vi "Car Wash Main.vi"() -> ()   [LabVIEW 2018]
doc: "The Car Wash Main VI is the main application that will provide the user with the interactive interface to initiate a car wash. This VI will utilize JKI state machine to incorperate each state of the car wash."
uses:
  Controls/Wash Option.ctl
  Controls/Wash Option Indicators.ctl
  Controls/Car Position.ctl
panel:
  in  "Car Position Slider":T1 scale=0.0..4.0
  out "Elapse Time":dbl format="%#_3g"
  in  "Stop Program":bool
  out "Wash Entry":bool
  out "Car Wash Indicators":T2
  in  "Start":bool
  in  "Wash Option":T3
  # "Entry Console"
  # "Car Wash Display"
  # "Pre-Soak\nH-P Wash\nL-P Waxx\nSpot Free Rinse"
  # "Underbody Wash\nBug Remover"
  # "Tire Shine\nAir Dry"
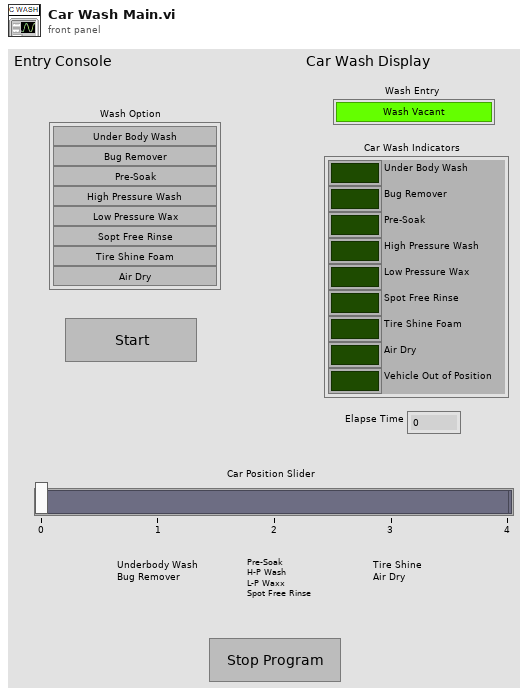
[diagram p1: front panel]
types:
  T1 = typedef "Car Position.ctl" = i32
  T2 = typedef "Wash Option Indicators.ctl" = cluster{"Under Body Wash":bool, "Bug Remover":bool, "Pre-Soak":bool, "High Pressure Wash":bool, "Low Pressure Wax":bool, "Spot Free Rinse":bool, "Tire Shine Foam":bool, "Air Dry":bool, "Vehicle Out of Position":bool}
  T3 = typedef "Wash Option.ctl" = cluster{"Under Body Wash":bool, "Bug Remover":bool, "Pre-Soak":bool, "High Pressure Wash":bool, "Low Pressure Wax":bool, "Spot Free Rinse":bool, "Tire Shine Foam":bool, "Air Dry":bool}
  T4 = enum32{"Invalid", "Standard", "Closed", "Hidden", "Minimized", "Maximized"}
  T5 = enum32{"invalid app kind", "Development System", "Run Time System", "Student Edition", "Embedded LabVIEW", "Evaluation", "Custom"}
  T6 = cluster{"Core":cluster{"Current VI Reference":refnum<vi>, "Close Panel on Exit?":bool}, "Current Car Wash Remaining":bool[], "Car Current Position":T1, "Current Elapse Time":dbl, "Start Time":timestamp, "Start Wash":bool, "Current Wash Index":i32}
  T7 = cluster{"Current VI Reference":refnum<vi>, "Close Panel on Exit?":bool}
  T8 = enum8{"Enabled", "Disabled", "Disabled and Grayed Out"}
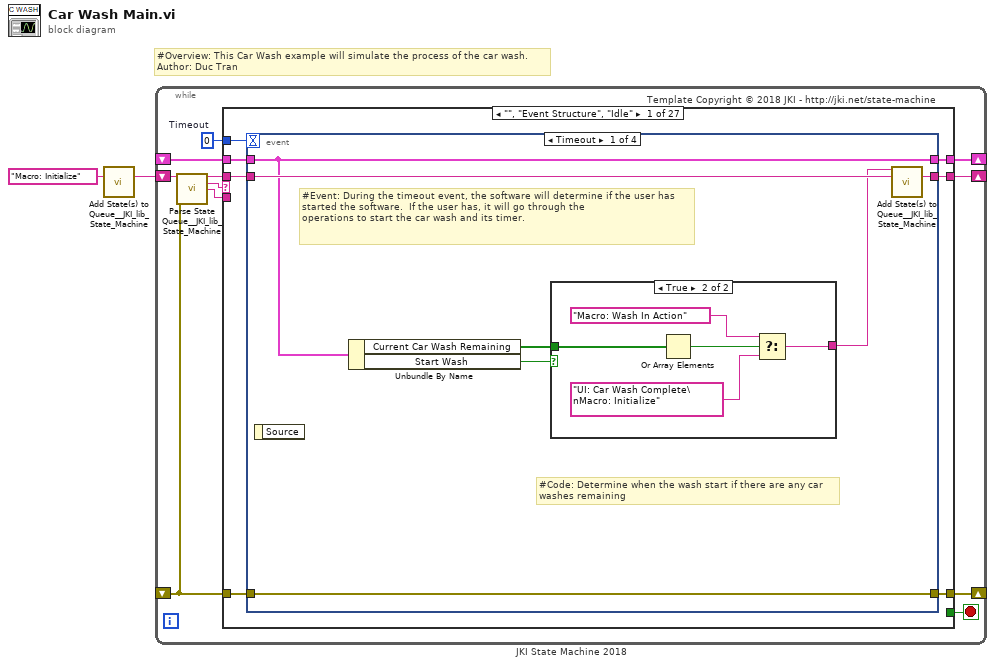
[diagram p0: block diagram]
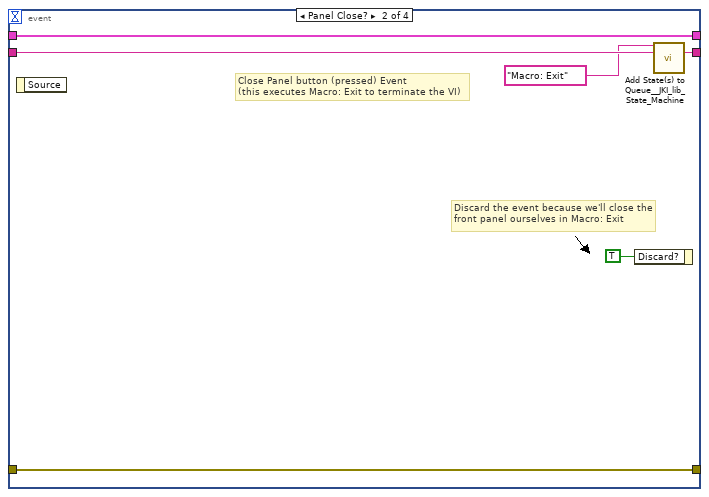
[diagram p3: hidden frame]
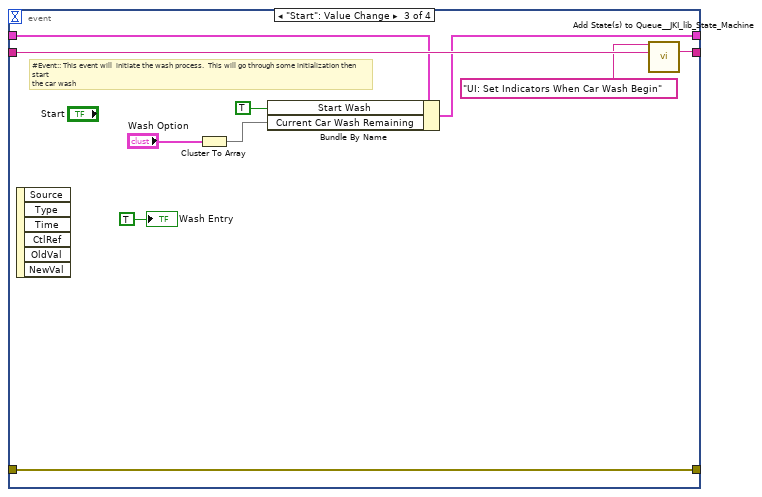
[diagram p4: hidden frame]
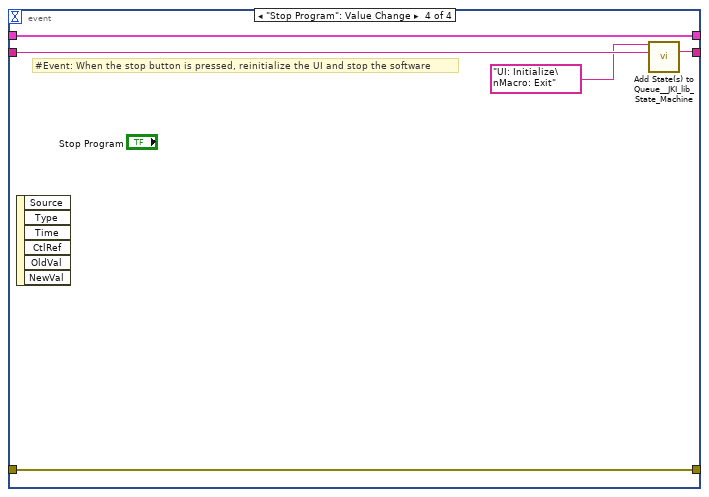
[diagram p5: hidden frame]
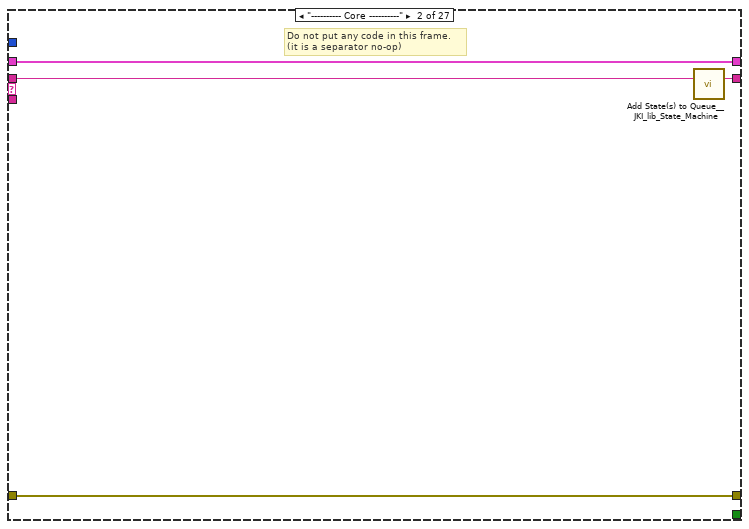
[diagram p6: hidden frame]
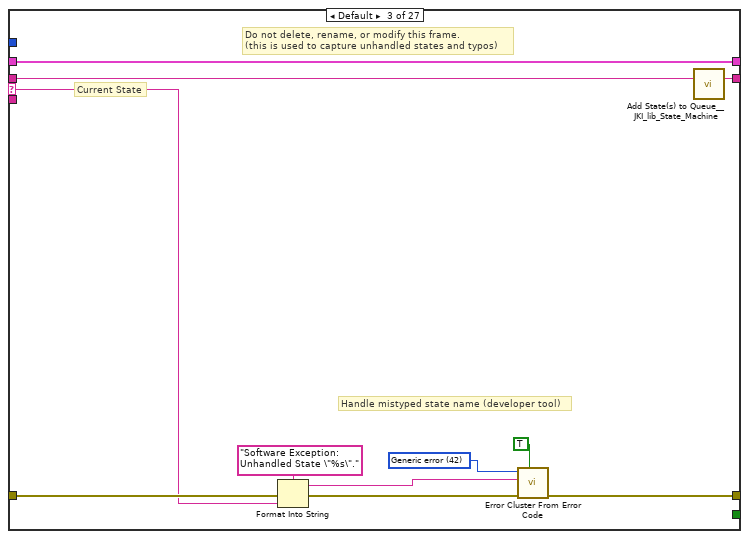
[diagram p7: hidden frame]
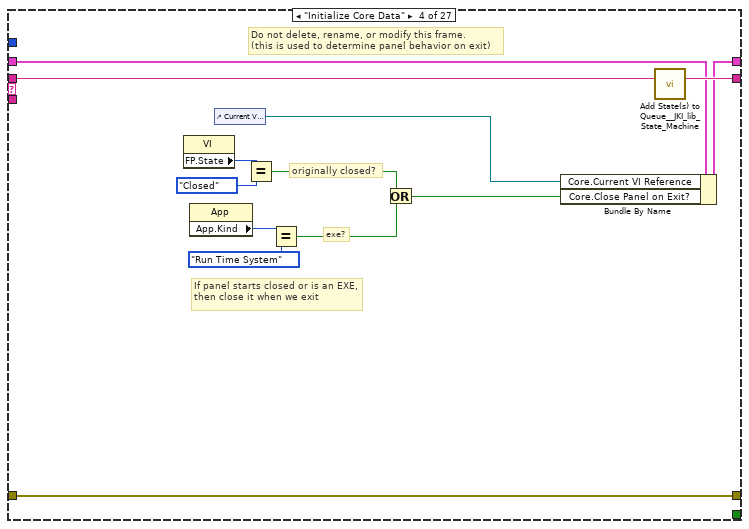
[diagram p8: hidden frame]
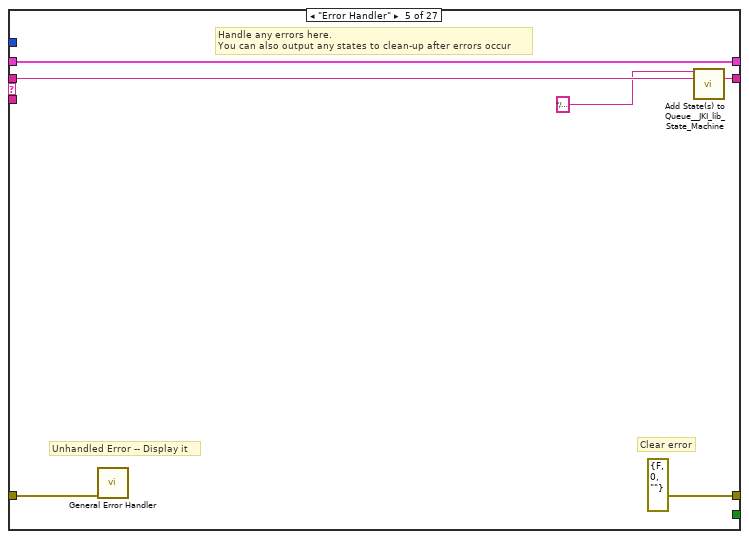
[diagram p9: hidden frame]
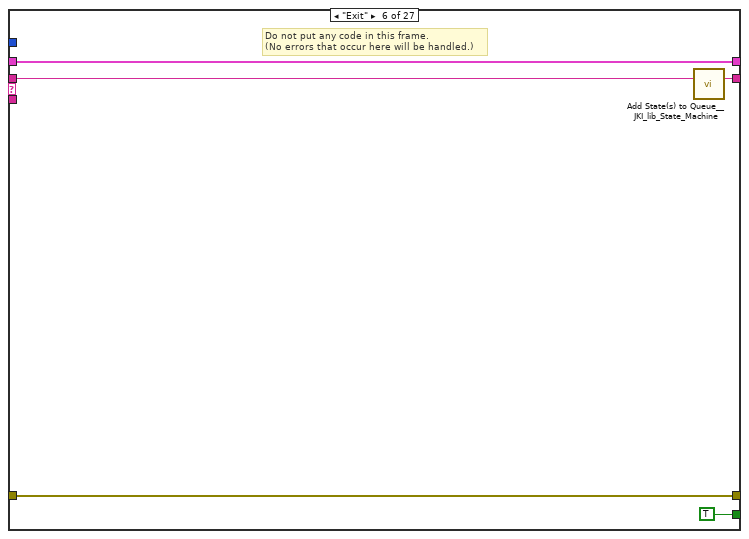
[diagram p10: hidden frame]
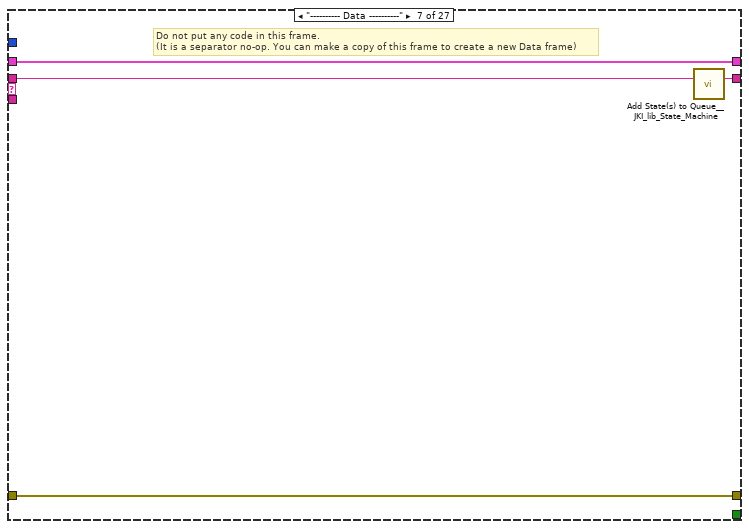
[diagram p11: hidden frame]
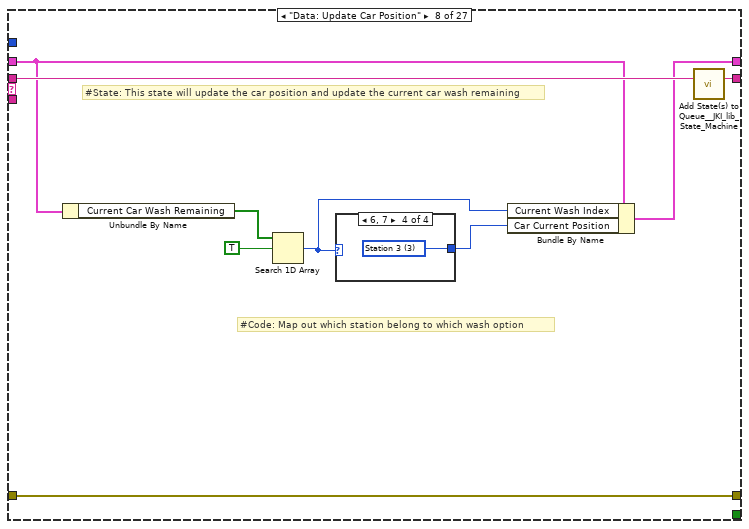
[diagram p12: hidden frame]
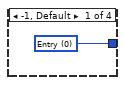
[diagram p13: hidden frame]
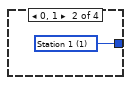
[diagram p14: hidden frame]
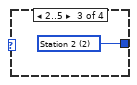
[diagram p15: hidden frame]
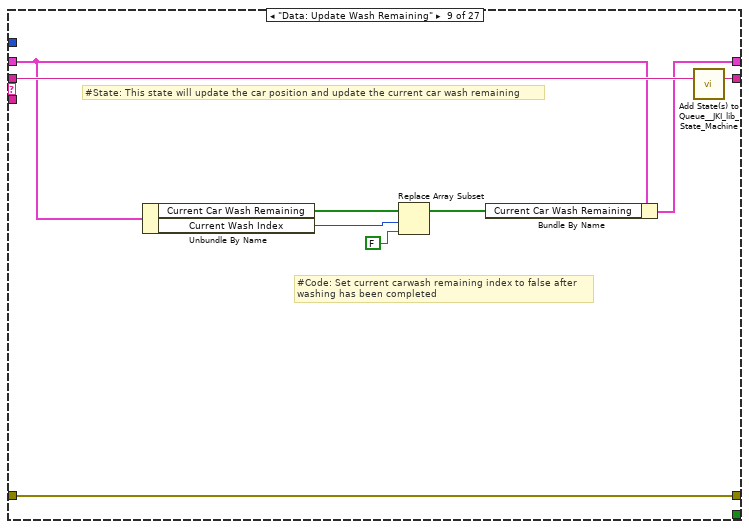
[diagram p16: hidden frame]
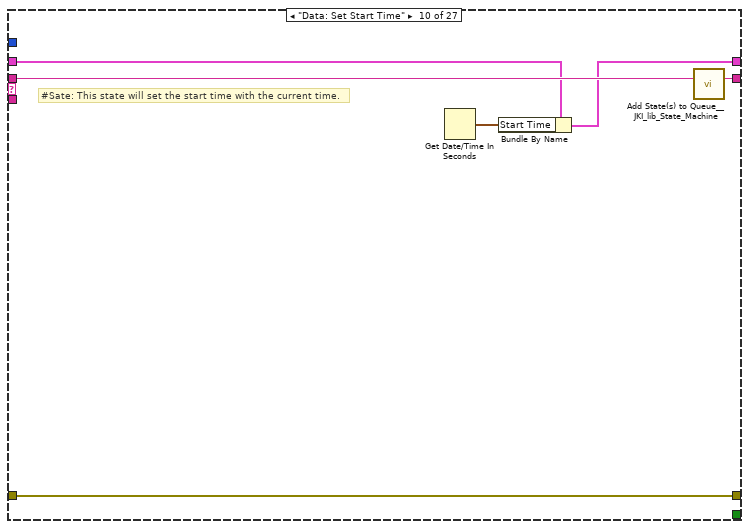
[diagram p17: hidden frame]
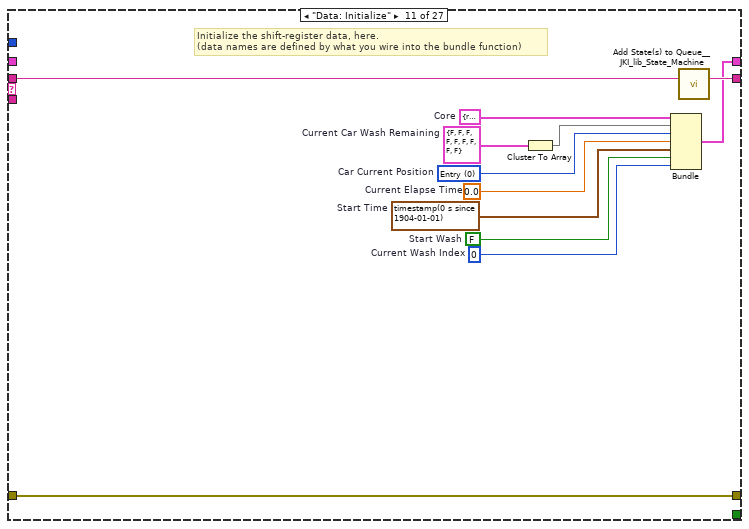
[diagram p18: hidden frame]
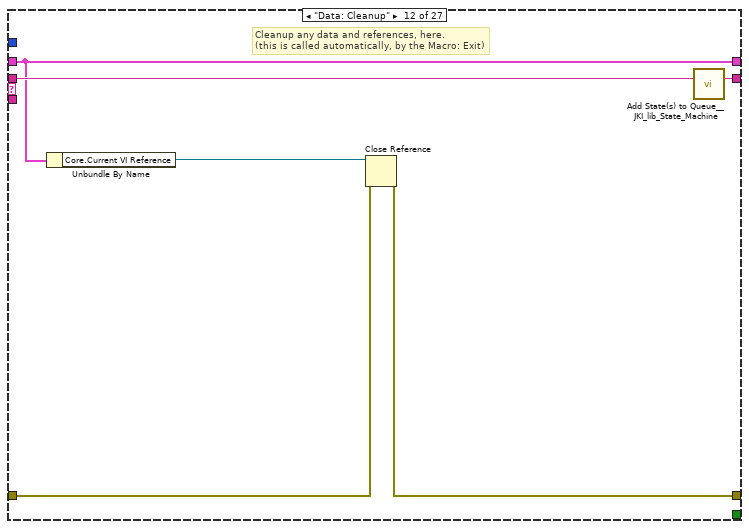
[diagram p19: hidden frame]
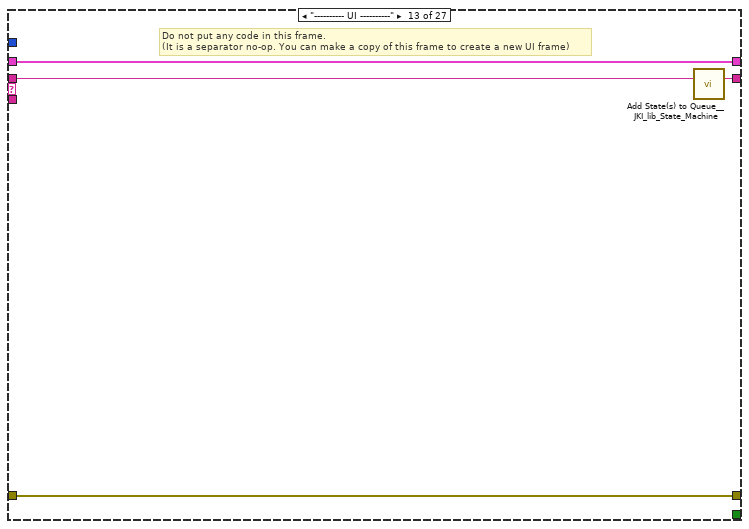
[diagram p20: hidden frame]
diagram:
  # "#Overview: This Car Wash example will simulate the process of the car wash.\nAuthor: Duc Tran"
  n1 = call <vilib>:"Add State(s) to Queue__JKI_lib_State_Machine.vi"("State(s) in (\"\")"="Macro: Initialize") -> ("States Out"=w1:string)  [unwired: 14 in]
  n2 = while "JKI State Machine 2018" {
    shift-right: [w6] -> _
    shift-left: _ -> [w5]
    shift-right: [w9] -> _
    shift-left: _ -> [w3]
    shift-right: [w8] -> _
    shift-left: w1 -> [w10]
    stop <- w7 stop-if-true
    w4 = 0  # Timeout
    # "Template Copyright © 2018 JKI - http://jki.net/state-machine"
    n3 = call <vilib>:"Parse State Queue__JKI_lib_State_Machine.vi"("State Queue"=w10, "Error In (no error)"=w3) -> ("Remaining States"=w12:string, "Current State"=w13:string, "Arguments"=w11:string)  [unwired: 11 in]
    n4 = case shown="\"\", \"Event Structure\", \"Idle\"" w13 {
      selector: w13 -> [_ _ w58 _ _ _ _ _ _ _ _ _ _ _ _ _ _ _ _ _ _ _ _ _ _ _ _]
      tunnel: w12 -> [w20 w57 w62 w81 w87 w92 w96 w105 w118 w124 w136 w142 w146 w149 w172 w179 w185 w200 w206 w217 w286 w291 w296 w306 w310 w320 w340]
      tunnel: w11 -> [_ _ _ _ _ _ _ _ _ _ _ _ _ _ _ _ _ _ w201 w211 _ _ _ _ _ _ _]
      tunnel: w5 -> [w18 w54 w60 w74 w84 w90 w93 w100 w115 w121 _ w138 w143 w150 w171 w177 w186 w198 w204 w213 w283 w288 w293 w303 w307 w317 w333]
      tunnel: [w17 w55 w64 w78 errorcluster {"status"=FALSE, "code"=0, "source"=""} ("error out") w89 w94 w103 w116 w122 w133 w139 w144 w151 w173 w180 w181 w189 w202 w214 w284 w289 w294 w304 w308 w318 w338] -> w9
      tunnel: w3 -> [w16 w55 w63 w78 w83 w89 w94 w103 w116 w122 w133 w137 w144 w151 w173 w180 w182 w194 w203 w215 w284 w289 w294 w304 w308 w318 w338]
      tunnel: [w19 w56 w61 w80 w86 w91 w95 w104 w117 w123 w135 w141 w145 w149 w172 w179 w185 w199 w205 w216 w285 w290 w295 w305 w309 w319 w339] -> w8
      tunnel: [_ _ _ _ _ TRUE _ _ _ _ _ _ _ _ _ _ _ _ _ _ _ _ _ _ _ _ _] -> w7
      tunnel: [w15 w54 w60 w79 w84 w90 w93 w99 w114 w120 w134 w138 w143 w150 w171 w175 w186 w198 w204 w213 w283 w288 w293 w303 w307 w317 w331] -> w6
      tunnel: w4 -> [w14 _ _ _ _ _ _ _ _ _ _ _ _ _ _ _ _ _ _ _ _ _ _ _ _ _ _]
      frame "", "Event Structure", "Idle" {
        n5 = event shown="[0] Timeout" {
          selector: _ -> [_ _ _ _]
          dyn-events: _ -> [_ _ _ _]
          timeout: w14 -> [_ _ _ _]
          tunnel: w20 -> [w27 w38 w48 w52]
          tunnel: [w26 w37 w47 w51] -> w19
          tunnel: w18 -> [w24 w35 w44 w53]
          tunnel: [w25 w36 w45 w49] -> w17
          tunnel: w16 -> [w25 w36 w45 w49]
          tunnel: [w24 w35 w42 w53] -> w15
          event Timeout {
            # "#Code: Determine when the wash start if there are any car\nwashes remaining"
            # "#Event: During the timeout event, the software will determine if the user has started the software.  If the user has, it will go through the\noperations to start the car wash and its timer."
            n6 = event-data() -> ()  [unwired: 1 in, 1 out]
            n7 = Unbundle By Name(w24) -> ("Current Car Wash Remaining"=w22:bool[], "Start Wash"=w23:bool)
            n8 = case shown="True" w23 {
              tunnel: w22 -> [_ w28]
              tunnel: [_ w30] -> w21
              frame False {
              }
              frame True {
                n9 = Or Array Elements(Boolean array=w28) -> (logical OR=w32:bool)
                n10 = Select(t="Macro: Wash In Action", s=w32, f="UI: Car Wash Complete\nMacro: Initialize") -> (s? t:f=w30:string)
              }
            }
            n11 = call <vilib>:"Add State(s) to Queue__JKI_lib_State_Machine.vi"("State(s) in Front (\"\")"=w21, "State(s) in (\"\")"=w27) -> ("States Out"=w26:string)  [unwired: 13 in]
          }
          event Panel Close? {
            # "Discard the event because we'll close the front panel ourselves in Macro: Exit"
            # "Close Panel button (pressed) Event\n(this executes Macro: Exit to terminate the VI)"
            n12 = event-data() -> ()  [unwired: 1 in, 1 out]
            n13 = event-data("Discard?"=TRUE) -> ()  [unwired: 1 in, 1 out]
            n14 = call <vilib>:"Add State(s) to Queue__JKI_lib_State_Machine.vi"("State(s) in Front (\"\")"="Macro: Exit", "State(s) in (\"\")"=w38) -> ("States Out"=w37:string)  [unwired: 13 in]
          }
          event "Start": Value Change {
            # "#Event:: This event will  initiate the wash process.  This will go through some initialization then start\nthe car wash"
            n15 = event-data() -> ()  [unwired: 1 in, 6 out]
            n16 = Cluster To Array(cluster="Wash Option") -> (array=w40:bool[])
            n17 = Bundle By Name(cluster=w44, "Start Wash"=TRUE, "Current Car Wash Remaining"=w40) -> (w42:T6)
            n18 = call <vilib>:"Add State(s) to Queue__JKI_lib_State_Machine.vi"("State(s) in Front (\"\")"="UI: Set Indicators When Car Wash Begin", "State(s) in (\"\")"=w48) -> ("States Out"=w47:string)  [unwired: 13 in]
            "Wash Entry" <- TRUE ("Wash Entry")
          }
          event "Stop Program": Value Change {
            # "#Event: When the stop button is pressed, reinitialize the UI and stop the software"
            n19 = event-data() -> ()  [unwired: 1 in, 6 out]
            n20 = call <vilib>:"Add State(s) to Queue__JKI_lib_State_Machine.vi"("State(s) in Front (\"\")"="UI: Initialize\nMacro: Exit", "State(s) in (\"\")"=w52) -> ("States Out"=w51:string)  [unwired: 13 in]
          }
        }
      }
      frame "---------- Core ----------" {
        # "Do not put any code in this frame.\n(it is a separator no-op)"
        n21 = call <vilib>:"Add State(s) to Queue__JKI_lib_State_Machine.vi"("State(s) in (\"\")"=w57) -> ("States Out"=w56:string)  [unwired: 14 in]
      }
      frame Default {
        w67 = 42 items=["No error", "Argument error", "Memory is full", "Out of zone", "End of file", "File already open", "Generic file I/O error", "File not found", "File permission error", "Disk is full", "Duplicate path", "Too many files open", "System feature not enabled", "Resource file not found", "Cannot add resource", "Resource not found", "Image not found", "Image memory error", "Pen does not exist", "Config type invalid", "Config token not found", "Config parse error", "Config memory error", "Bad external code format", "Bad external code offset", "External code not present", "Null window", "Destroy window error", "Null menu", "Print aborted", "Bad print record", "Print driver error", "Windows error during printing", "Memory error during printing", "Print dialog error", "Generic print error", "Invalid device refnum", "Device not found", "Device parameter error", "Device unit error", "Cannot open device", "Device call aborted", "Generic error", "Cancelled by user", "Object ID too low", "Object ID too high", "Object not in heap", "Unknown heap", "Unknown object (invalid DefProc)", "Unknown object (DefProc not in table)", "Message out of range", "Invalid (null) method", "Unknown message", "Manager call not supported", "Bad address", "Network operation in progress", "Network operation timed out", "Connection is busy", "Network attribute not supported", "Network error", "Address in use", "System out of memory", "Connection aborted", "Connection refused", "Not connected", "Already connected", "Connection closed", "Initialization error (interapplication manager)", "Bad occurrence", "Wait on unbound occurrence handler", "Occurrence queue overflow", "Datalog type conflict", "Unused", "Unrecognized type (interapplication manager)", "Memory corrupt", "Failed to make temporary DLL", "Old CIN version", "Drag socket not found", "Failed to load drop-object", "Failed to register OLE object", "Failed to release OLE object", "Format specifier type mismatch", "Unknown format specifier", "Too few format specifiers", "Too many format specifiers", "Scan failed", "Newer CIN version", "Error converting to variant", "Runtime menu error", "Password tampered", "Variant attribute not found", "Incompatible variant data type", "Event data is not available", "Event Store is not present", "Occurrence is not found", "Event Queue is not created", "Event info is not available", "Refnum passed is NULL", "Error retrieving Class GUID", "Error retrieving CoClass GUID", "Error retrieving TypeLib GUID.", "Bad built application magic bytes.", "Specific driver is different from the specific driver associated with the Logical Name.", "There is no session opened to the class driver.", "Max Error", "MAX - Error with config objects", "MAX - Error loading configuration", "MAX - Group not supported"]
        # "Current State"
        # "Do not delete, rename, or modify this frame.\n(this is used to capture unhandled states and typos)"
        # "Handle mistyped state name (developer tool)"
        n22 = Format Into String(format string="Software Exception: Unhandled State \"%s\"." ("message"), error in=w63, w58) -> (resulting string=w66:string, error out=w65:errorcluster)  [unwired: 1 in]
        n23 = call <vilib>:"Error Cluster From Error Code.vi"("show call chain? (False)"=TRUE, "error in (no error)"=w65, "error message (\"\")"=w66, "error code (0)"=w67) -> ("error out"=w64:errorcluster)  [unwired: 5 in]
        n24 = call <vilib>:"Add State(s) to Queue__JKI_lib_State_Machine.vi"("State(s) in (\"\")"=w62) -> ("States Out"=w61:string)  [unwired: 14 in]
      }
      frame "Initialize Core Data" {
        # "Do not delete, rename, or modify this frame.\n(this is used to determine panel behavior on exit)"
        # "originally closed?"
        # "exe?"
        # "If panel starts closed or is an EXE, then close it when we exit"
        n25 = property class="VI"() -> ("FP.State"=w71:T4)  [unwired: 2 in, 2 out]
        n26 = property class="App"() -> ("App.Kind"=w77:T5)  [unwired: 2 in, 2 out]
        n27 = control-ref of="Current VI Reference"() -> (w72:refnum<vi>)
        n28 = Equal?(x=w71, y=T4."Closed" ("Front Panel Window:State")) -> (x = y?=w69:bool)
        n29 = Equal?(x=w77, y=T5."Run Time System" ("Application:Kind")) -> (x = y?=w75:bool)
        n30 = Or(x=w69, y=w75) -> (x .or. y?=w73:bool)
        n31 = Bundle By Name(cluster=w74, "Core.Current VI Reference"=w72, "Core.Close Panel on Exit?"=w73) -> (w79:T6)
        n32 = call <vilib>:"Add State(s) to Queue__JKI_lib_State_Machine.vi"("State(s) in (\"\")"=w81) -> ("States Out"=w80:string)  [unwired: 14 in]
      }
      frame "Error Handler" {
        # "Unhandled Error -- Display it"
        # "Handle any errors here.\nYou can also output any states to clean-up after errors occur"
        # "Clear error"
        n33 = call <vilib>:"General Error Handler.vi"("error in (no error)"=w83) -> ()  [unwired: 10 in, 5 out]
        n34 = call <vilib>:"Add State(s) to Queue__JKI_lib_State_Machine.vi"("State(s) in Front (\"\")"="/* Post Error States", "State(s) in (\"\")"=w87) -> ("States Out"=w86:string)  [unwired: 13 in]
      }
      frame "Exit" {
        # "Do not put any code in this frame.\n(No errors that occur here will be handled.)"
        n35 = call <vilib>:"Add State(s) to Queue__JKI_lib_State_Machine.vi"("State(s) in (\"\")"=w92) -> ("States Out"=w91:string)  [unwired: 14 in]
      }
      frame "---------- Data ----------" {
        # "Do not put any code in this frame.\n(It is a separator no-op. You can make a copy of this frame to create a new Data frame)"
        n36 = call <vilib>:"Add State(s) to Queue__JKI_lib_State_Machine.vi"("State(s) in (\"\")"=w96) -> ("States Out"=w95:string)  [unwired: 14 in]
      }
      frame "Data: Update Car Position" {
        # "#Code: Map out which station belong to which wash option"
        # "#State: This state will update the car position and update the current car wash remaining"
        n37 = Unbundle By Name(w100) -> ("Current Car Wash Remaining"=w101:bool[])
        n38 = Search 1D Array(1D array=w101, element=TRUE) -> (index of element=w97:i32)  [unwired: 1 in]
        n39 = case shown="6, 7" w97 {
          tunnel: [w106 w107 w108 w109] -> w98
          frame -1, Default {
            w106 = T1 0 items=["Entry", "Station 1", "Station 2", "Station 3", "Exit"] ("Car Current Position")
          }
          frame 0, 1 {
            w107 = T1 1 items=["Entry", "Station 1", "Station 2", "Station 3", "Exit"] ("Car Current Position")
          }
          frame 2..5 {
            w108 = T1 2 items=["Entry", "Station 1", "Station 2", "Station 3", "Exit"] ("Car Current Position")
          }
          frame 6, 7 {
            w109 = T1 3 items=["Entry", "Station 1", "Station 2", "Station 3", "Exit"] ("Car Current Position")
          }
        }
        n40 = Bundle By Name(cluster=w100, "Current Wash Index"=w97, "Car Current Position"=w98) -> (w99:T6)
        n41 = call <vilib>:"Add State(s) to Queue__JKI_lib_State_Machine.vi"("State(s) in (\"\")"=w105) -> ("States Out"=w104:string)  [unwired: 14 in]
      }
      frame "Data: Update Wash Remaining" {
        # "#Code: Set current carwash remaining index to false after\nwashing has been completed"
        # "#State: This state will update the car position and update the current car wash remaining"
        n42 = Unbundle By Name(w115) -> ("Current Car Wash Remaining"=w112:bool[], "Current Wash Index"=w111:i32)
        n43 = Replace Array Subset(array=w112, new element=FALSE ("element"), index=w111) -> (w110:bool[])
        n44 = Bundle By Name(cluster=w115, "Current Car Wash Remaining"=w110) -> (w114:T6)
        n45 = call <vilib>:"Add State(s) to Queue__JKI_lib_State_Machine.vi"("State(s) in (\"\")"=w118) -> ("States Out"=w117:string)  [unwired: 14 in]
      }
      frame "Data: Set Start Time" {
        # "#Sate: This state will set the start time with the current time."
        n46 = Get Date/Time In Seconds() -> (seconds since 1Jan1904=w119:timestamp)
        n47 = Bundle By Name(cluster=w121, "Start Time"=w119) -> (w120:T6)
        n48 = call <vilib>:"Add State(s) to Queue__JKI_lib_State_Machine.vi"("State(s) in (\"\")"=w124) -> ("States Out"=w123:string)  [unwired: 14 in]
      }
      frame "Data: Initialize" {
        w125 = timestamp(0 s since 1904-01-01)  # Start Time
        w126 = 0  # Current Wash Index
        w128 = T2 {"Under Body Wash"=FALSE, "Bug Remover"=FALSE, "Pre-Soak"=FALSE, "High Pressure Wash"=FALSE, "Low Pressure Wax"=FALSE, "Spot Free Rinse"=FALSE, "Tire Shine Foam"=FALSE, "Air Dry"=FALSE, "Vehicle Out of Position"=FALSE}  # Current Car Wash Remaining
        w129 = FALSE  # Start Wash
        w130 = 0.0  # Current Elapse Time
        w131 = T1 0 items=["Entry", "Station 1", "Station 2", "Station 3", "Exit"]  # Car Current Position
        w132 = T7 {"Current VI Reference"=refnum, "Close Panel on Exit?"=FALSE}  # Core
        # "Initialize the shift-register data, here.\n(data names are defined by what you wire into the bundle function)"
        n49 = Cluster To Array(cluster=w128) -> (array=w127:bool[])
        n50 = Bundle("Core"=w132, "Current Car Wash Remaining"=w127, "Car Current Position"=w131, "Current Elapse Time"=w130, "Start Time"=w125, "Start Wash"=w129, "Current Wash Index"=w126) -> (w134:T6)  [unwired: 1 in]
        n51 = call <vilib>:"Add State(s) to Queue__JKI_lib_State_Machine.vi"("State(s) in (\"\")"=w136) -> ("States Out"=w135:string)  [unwired: 14 in]
      }
      frame "Data: Cleanup" {
        # "Cleanup any data and references, here.\n(this is called automatically, by the Macro: Exit)"
        n52 = Unbundle By Name(w138) -> ("Core.Current VI Reference"=w140:refnum<vi>)
        n53 = Close Reference(reference=w140, error in (no error)=w137) -> (error out=w139:errorcluster)
        n54 = call <vilib>:"Add State(s) to Queue__JKI_lib_State_Machine.vi"("State(s) in (\"\")"=w142) -> ("States Out"=w141:string)  [unwired: 14 in]
      }
      frame "---------- UI ----------" {
        # "Do not put any code in this frame.\n(It is a separator no-op. You can make a copy of this frame to create a new UI frame)"
        n55 = call <vilib>:"Add State(s) to Queue__JKI_lib_State_Machine.vi"("State(s) in (\"\")"=w146) -> ("States Out"=w145:string)  [unwired: 14 in]
      }
      frame "UI: Update Indicator for Car Not Station" {
        # "#State: When the user is on a station that is vacant, this state will sent all of the inidcators to its vacant state."
        n56 = local write "Car Wash Indicators"(T2 {"Under Body Wash"=FALSE, "Bug Remover"=FALSE, "Pre-Soak"=FALSE, "High Pressure Wash"=FALSE, "Low Pressure Wax"=FALSE, "Spot Free Rinse"=FALSE, "Tire Shine Foam"=FALSE, "Air Dry"=FALSE, "Vehicle Out of Position"=TRUE} ("Car Wash Indicators")) -> ()
        n57 = local write "Elapse Time"(0.0 ("Elapse Time")) -> ()
      }
      frame "UI: Update Indicator for Car in Station" {
        # "#Code: Determine the carwash indication output.  this will output the LED indicator based\non the was that is currently taking place"
        # "#State: When the  station is not vacant, this state will set the indicators to the non vacant state."
        n58 = Unbundle By Name(w171) -> ("Current Elapse Time"=→"Elapse Time":dbl, "Current Car Wash Remaining"=w166:bool[], "Current Wash Index"=w153:i32)
        n59 = Array Size(array=w166) -> (size(s)=w165:i32)
        n60 = Initialize Array(FALSE, w165) -> (w164:bool[])
        n61 = Replace Array Subset(array=w164, new element=TRUE, index=w153) -> (w163:bool[])
        n62 = Index Array(array=w163) -> (element #1=w162:bool, element #2=w161:bool, element #3=w160:bool, element #4=w159:bool, element #5=w158:bool, element #6=w157:bool, element #7=w156:bool, element #8=w155:bool, element #9=w154:bool)  [unwired: 9 in]
        n63 = Bundle(cluster=T2 {"Under Body Wash"=FALSE, "Bug Remover"=FALSE, "Pre-Soak"=FALSE, "High Pressure Wash"=FALSE, "Low Pressure Wax"=FALSE, "Spot Free Rinse"=FALSE, "Tire Shine Foam"=FALSE, "Air Dry"=FALSE, "Vehicle Out of Position"=FALSE} ("Car Wash Indicators"), "Under Body Wash"=w162, "Bug Remover"=w161, "Pre-Soak"=w160, "High Pressure Wash"=w159, "Low Pressure Wax"=w158, "Spot Free Rinse"=w157, "Tire Shine Foam"=w156, "Air Dry"=w155, "Vehicle Out of Position"=w154) -> (→"Car Wash Indicators":T2)
      }
      frame "UI: Car Wash Complete" {
        w176 = T1 4 items=["Entry", "Station 1", "Station 2", "Station 3", "Exit"] ("Car Current Position")
        # "#Code: Once Car wash is completed\nset the car position to exit"
        # "#State: this complete message will fire when the car is finished with its wash conditions"
        n64 = local write "Wash Entry"(FALSE ("Wash Entry")) -> ()
        n65 = One Button Dialog(message="Car Wash Completed") -> ()  [unwired: 1 in, 1 out]
        n66 = Bundle By Name(cluster=w177, "Car Current Position"=w176) -> (w175:T6)
      }
      frame "UI: Set Indicators When Car Wash Begin" {
        w183 = T8."Disabled and Grayed Out" ("Disabled")
        # "#State: The start car wash UI event will set all of the events that needs to happen when the car wash begins.  This includes disabling the wash option and start control as well as enabling the stop control"
        n67 = property on="Wash Option" class="Clust"(error in=w182, "DisabledEnum"=w183) -> (error out=w184:errorcluster)  [unwired: 1 in, 1 out]
        n68 = property on="Start" class="Bool"(error in=w184, "DisabledEnum"=w183) -> (error out=w181:errorcluster)  [unwired: 1 in, 1 out]
      }
      frame "UI: Initialize" {
        w188 = T1 0 items=["Entry", "Station 1", "Station 2", "Station 3", "Exit"] ("Car Position Slider")
        w187 = T8."Enabled" ("Disabled")
        # "#State: This state will initialize all of the variable neccessary in the wash option of the software."
        # "Initialize the User Interface, here.\n(this is called automatically, by the Macro: Init)"
        n69 = property on="Wash Option" class="Clust"(error in=w194, "DisabledEnum"=w187) -> (error out=w193:errorcluster)  [unwired: 1 in, 1 out]
        n70 = property on="Start" class="Bool"(error in=w193, "DisabledEnum"=w187) -> (error out=w192:errorcluster)  [unwired: 1 in, 1 out]
        n71 = local write "Car Position Slider"(w188) -> ()
        n72 = local write "Car Wash Indicators"(T2 {"Under Body Wash"=FALSE, "Bug Remover"=FALSE, "Pre-Soak"=FALSE, "High Pressure Wash"=FALSE, "Low Pressure Wax"=FALSE, "Spot Free Rinse"=FALSE, "Tire Shine Foam"=FALSE, "Air Dry"=FALSE, "Vehicle Out of Position"=FALSE} ("Car Wash Indicators")) -> ()
        n73 = local write "Wash Entry"(FALSE ("Wash Entry")) -> ()
        n74 = local write "Elapse Time"(0.0 ("Elapse Time")) -> ()
        n75 = property on="Stop Program" class="Bool"(error in=w192, "DisabledEnum"=w187) -> (error out=w190:errorcluster)  [unwired: 1 in, 1 out]
        n76 = property on="Wash Option" class="Clust"(error in=w190, "Value"=T3 {"Under Body Wash"=FALSE, "Bug Remover"=FALSE, "Pre-Soak"=FALSE, "High Pressure Wash"=FALSE, "Low Pressure Wax"=FALSE, "Spot Free Rinse"=FALSE, "Tire Shine Foam"=FALSE, "Air Dry"=FALSE} ("Wash Option")) -> (error out=w189:errorcluster)  [unwired: 1 in, 1 out]
        n77 = call <vilib>:"Add State(s) to Queue__JKI_lib_State_Machine.vi"("State(s) in (\"\")"=w200) -> ("States Out"=w199:string)  [unwired: 14 in]
      }
      frame "UI: Cursor Set" {
        # "Argument"
        # "Set and Unset Cursor Busy.\n(Usage: \"UI: Cursor Set >> Busy|Idle\")"
        n78 = case shown="\"Idle\", Default" w201 {
          tunnel: w203 -> [w208 w210]
          tunnel: [w207 w209] -> w202
          frame "Idle", Default {
            n79 = call <vilib>:"Unset Busy.vi"("error in (no error)"=w208) -> ("error out"=w207:errorcluster)  [unwired: 10 in]
          }
          frame "Busy" {
            n80 = call <vilib>:"Set Busy.vi"("error in (no error)"=w210) -> ("error out"=w209:errorcluster)  [unwired: 9 in, 1 out]
          }
        }
        n81 = call <vilib>:"Add State(s) to Queue__JKI_lib_State_Machine.vi"("State(s) in (\"\")"=w206) -> ("States Out"=w205:string)  [unwired: 14 in]
      }
      frame "UI: Front Panel State" {
        # "Argument"
        # "Set Front Panel Open or Closed\n(Usage: \"UI: Front Panel State >> Open|Close\")"
        n82 = Unbundle By Name(w213) -> ("Core.Current VI Reference"=w212:refnum<vi>)
        n83 = case shown="\"Minimize\", \"Minimized\"" w211 {
          tunnel: w215 -> [w223 w238 w249 w262 w275]
          tunnel: [w225 w239 w251 w264 w277] -> w214
          tunnel: w212 -> [w224 w236 w250 w263 w276]
          frame "Open", "Standard", Default {
            w218 = T4."Standard" ("State")
            n84 = property class="VI"(reference=w224, error in=w223) -> (reference out=w221:refnum<vi>, error out=w222:errorcluster, "FP.State"=w220:T4)
            n85 = Not Equal?(x=w220, y=w218) -> (x != y?=w219:bool)
            n86 = case shown="True" w219 {
              tunnel: [w229 w231] -> w225
              tunnel: w222 -> [w228 w231]
              tunnel: w221 -> [w227 _]
              tunnel: w218 -> [w226 _]
              frame True {
                n87 = invoke class="VI" method="FP.Open"(reference=w227, error in=w228, "Activate"=TRUE, "State"=w226) -> (error out=w229:errorcluster)  [unwired: 1 in, 4 out]
              }
              frame False {
              }
            }
          }
          frame "Close", "Closed" {
            n88 = property class="VI"(reference=w236, error in=w238) -> (reference out=w235:refnum<vi>, error out=w237:errorcluster, "FP.State"=w233:T4)
            n89 = Not Equal?(x=w233, y=T4."Closed" ("Front Panel Window:State")) -> (x != y?=w232:bool)
            n90 = case shown="True" w232 {
              tunnel: [w240 w243] -> w239
              tunnel: w237 -> [w240 w242]
              tunnel: w235 -> [_ w241]
              frame False {
              }
              frame True {
                n91 = invoke class="VI" method="FP.Close"(reference=w241, error in=w242) -> (error out=w243:errorcluster)  [unwired: 1 in, 2 out]
              }
            }
          }
          frame "Hidden", "Hide" {
            w244 = T4."Hidden" ("State")
            n92 = property class="VI"(reference=w250, error in=w249) -> (reference out=w247:refnum<vi>, error out=w248:errorcluster, "FP.State"=w246:T4)
            n93 = Not Equal?(x=w246, y=w244) -> (x != y?=w245:bool)
            n94 = case shown="True" w245 {
              tunnel: [w255 w256] -> w251
              tunnel: w248 -> [w254 w256]
              tunnel: w247 -> [w253 _]
              tunnel: w244 -> [w252 _]
              frame True {
                n95 = invoke class="VI" method="FP.Open"(reference=w253, error in=w254, "State"=w252) -> (error out=w255:errorcluster)  [unwired: 2 in, 4 out]
              }
              frame False {
              }
            }
          }
          frame "Minimize", "Minimized" {
            w257 = T4."Minimized" ("State")
            n96 = property class="VI"(reference=w263, error in=w262) -> (reference out=w260:refnum<vi>, error out=w261:errorcluster, "FP.State"=w259:T4)
            n97 = Not Equal?(x=w259, y=w257) -> (x != y?=w258:bool)
            n98 = case shown="True" w258 {
              tunnel: [w268 w269] -> w264
              tunnel: w261 -> [w267 w269]
              tunnel: w260 -> [w266 _]
              tunnel: w257 -> [w265 _]
              frame True {
                n99 = invoke class="VI" method="FP.Open"(reference=w266, error in=w267, "State"=w265) -> (error out=w268:errorcluster)  [unwired: 2 in, 4 out]
              }
              frame False {
              }
            }
          }
          frame "Maximize", "Maximized" {
            w270 = T4."Maximized" ("State")
            n100 = property class="VI"(reference=w276, error in=w275) -> (reference out=w273:refnum<vi>, error out=w274:errorcluster, "FP.State"=w272:T4)
            n101 = Not Equal?(x=w272, y=w270) -> (x != y?=w271:bool)
            n102 = case shown="True" w271 {
              tunnel: [w281 w282] -> w277
              tunnel: w274 -> [w280 w282]
              tunnel: w273 -> [w279 _]
              tunnel: w270 -> [w278 _]
              frame True {
                n103 = invoke class="VI" method="FP.Open"(reference=w279, error in=w280, "State"=w278) -> (error out=w281:errorcluster)  [unwired: 2 in, 4 out]
              }
              frame False {
              }
            }
          }
        }
        n104 = call <vilib>:"Add State(s) to Queue__JKI_lib_State_Machine.vi"("State(s) in (\"\")"=w217) -> ("States Out"=w216:string)  [unwired: 14 in]
      }
      frame "---------- Macro ----------" {
        # "Do not put any code in this frame.\n(It is a separator no-op. You can make a copy of this frame to create a new Macro frame)"
        n105 = call <vilib>:"Add State(s) to Queue__JKI_lib_State_Machine.vi"("State(s) in (\"\")"=w286) -> ("States Out"=w285:string)  [unwired: 14 in]
      }
      frame "Macro: Wash In Action" {
        # "#State: This macro will launch when there is a wash in action.\nThis will go through the individual states to determine the current state, elapse time, etc."
        n106 = call <vilib>:"Add State(s) to Queue__JKI_lib_State_Machine.vi"("State(s) in Front (\"\")"="Decision: Elapse Time Five Seconds or Greater\nDecision: Car in Position", "State(s) in (\"\")"=w291) -> ("States Out"=w290:string)  [unwired: 13 in]
      }
      frame "Macro: Initialize" {
        w292 = "Data: Initialize\nInitialize Core Data\nUI: Initialize\nUI: Front Panel State >> Open"  # Data: Initialize Initialize Core Data UI: Initialize UI: Front Panel State >> Open
        # "Initialization Macro\n(This is called once, when the VI starts)"
        n107 = call <vilib>:"Add State(s) to Queue__JKI_lib_State_Machine.vi"("State(s) in Front (\"\")"=w292, "State(s) in (\"\")"=w296) -> ("States Out"=w295:string)  [unwired: 13 in]
      }
      frame "Macro: Exit" {
        # "Exit Macro\n(This is called once, when the VI exits)"
        n108 = Unbundle By Name(w303) -> ("Core.Close Panel on Exit?"=w302:bool)
        n109 = Select(t="UI: Front Panel State >> Close", s=w302, f="") -> (s? t:f=w299:string)
        n110 = call <vilib>:"Add State(s) to Queue__JKI_lib_State_Machine.vi"("State(s) in (\"\")"=w299, "State(s) at Back (\"\")"="Data: Cleanup\nExit") -> ("States Out"=w297:string)  [unwired: 13 in]
        n111 = call <vilib>:"Add State(s) to Queue__JKI_lib_State_Machine.vi"("State(s) in Front (\"\")"=w297, "State(s) in (\"\")"=w306) -> ("States Out"=w305:string)  [unwired: 13 in]
      }
      frame "---------- Decision ----------" {
        # "Template Separator\n(You can make a copy of, or modify, this frame)"
        n112 = call <vilib>:"Add State(s) to Queue__JKI_lib_State_Machine.vi"("State(s) in (\"\")"=w310) -> ("States Out"=w309:string)  [unwired: 14 in]
      }
      frame "Decision: Car in Position" {
        # "#State: This decision state will determine if the slider is currentlny in the position that the car is in.  If the slider is in the car's current position, then update the indicators with the updated value, else, update the indicator with the vacant indicator."
        n113 = Unbundle By Name(w317) -> ("Car Current Position"=w316:T1)
        n114 = Equal?(x=w316, y="Car Position Slider") -> (x = y?=w314:bool)
        n115 = Select(t="UI: Update Indicator for Car in Station", s=w314, f="UI: Update Indicator for Car Not Station") -> (s? t:f=w311:string)
        n116 = call <vilib>:"Add State(s) to Queue__JKI_lib_State_Machine.vi"("State(s) in Front (\"\")"=w311, "State(s) in (\"\")"=w320) -> ("States Out"=w319:string)  [unwired: 13 in]
      }
      frame "Decision: Elapse Time Five Seconds or Greater" {
        w321 = timestamp(0 s since 1904-01-01)  # Null Start
        # "#Code: If the Car Wash session just begin or\nthe time has elapsed."
        # "#Code: Format the update wash\nremaining into the queue"
        # "#Code: If another car wash session starts"
        # "#State: If the Elapse time is five seconds or greater, then go to the next operation"
        n117 = Unbundle By Name(w333) -> ("Start Time"=w322:timestamp)
        n118 = Get Date/Time In Seconds() -> (seconds since 1Jan1904=w335:timestamp)
        n119 = Subtract(x=w335, y=w322) -> (x-y=w332:dbl)
        n120 = Greater Or Equal?(x=w332, y=5.0) -> (x >= y?=w325:bool)
        n121 = Equal?(x=w321, y=w322) -> (x = y?=w323:bool)
        n122 = Or(x=w323, y=w325) -> (x .or. y?=w324:bool)
        n123 = Select(t="", s=w323, f=" Data: Update Wash Remaining") -> (s? t:f=w327:string)
        n124 = Format Into String(format string="%s\nData: Update Car Position\nData: Set Start Time", w327) -> (resulting string=w326:string)  [unwired: 2 in, 1 out]
        n125 = Bundle By Name(cluster=w333, "Current Elapse Time"=w332) -> (w331:T6)
        n126 = Select(t=w326, s=w324, f="") -> (s? t:f=w336:string)
        n127 = call <vilib>:"Add State(s) to Queue__JKI_lib_State_Machine.vi"("State(s) in Front (\"\")"=w336, "State(s) in (\"\")"=w340) -> ("States Out"=w339:string)  [unwired: 13 in]
      }
    }
  }
